vi "Extract last queue element.vi"(4 "Queue array in":T1[](array[typedef]) {"Initial time [s]" format="%_19f"; "Raw data [V]\n(all samples)" format="%0.2f"; "Timestamp [s]" format="%_19f"}) -> (0 "Loop count":i64, 1 "Queue array out":T1[](array[typedef]) {"Initial time [s]" format="%_19f"; "Raw data [V]\n(all samples)" format="%0.2f"; "Timestamp [s]" format="%_19f"}, 2 "Initial time":dbl)   [LabVIEW 2020]
uses:
  Queue.ctl
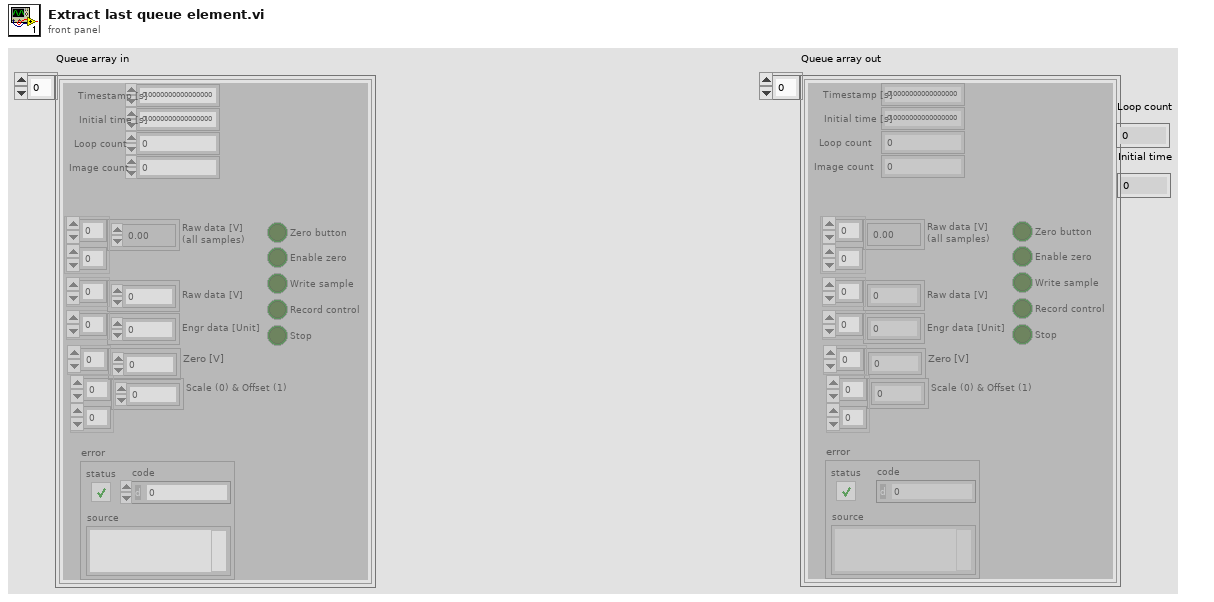
[diagram p1: front panel]
types:
  T1 = typedef "Queue.ctl" = cluster{"Enable zero":bool, "Engr data [Unit]":dbl[], "Zero button":bool, "Zero [V]":dbl[], "Timestamp [s]":dbl, "Write sample":bool, "Record control":bool, "Stop":bool, "error":errorcluster, "Raw data [V]\n(all samples)":dbl[][], "Raw data [V]":dbl[], "Loop count":i64, "Initial time [s]":dbl, "Scale (0) & Offset (1)":dbl[][], "Image count":dbl}
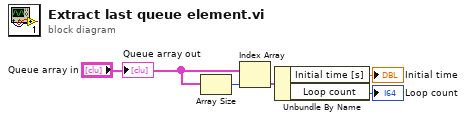
[diagram p0: block diagram]
diagram:
  n1 = Array Size(array="Queue array in") -> (size(s)=w5:i32)
  n2 = Index Array(array="Queue array in", index=w5) -> (element=w4:T1)
  n3 = Unbundle By Name(w4) -> ("Initial time [s]"=→"Initial time":dbl, "Loop count"=→"Loop count":i64)
  "Queue array out" <- "Queue array in"
